vi "PS_SET_VOLTAGE.vi"(0 "VISA resource name":refnum<visa-resource-name>, 1 "SEL_PS":string(combo), 2 "Skip(T)":bool, 11 "error in (no error)":errorcluster {"code" format="%.0x"}, 12 "Use Channel":bool[](array[boolean])=[TRUE, FALSE, FALSE, FALSE], 14 "Voltage Set":sgl[](array[numeric])) -> (4 "VISA resource name out":refnum<visa-resource-name>, 15 "error out":errorcluster {"code" format="%.0x"})   [LabVIEW 2018]
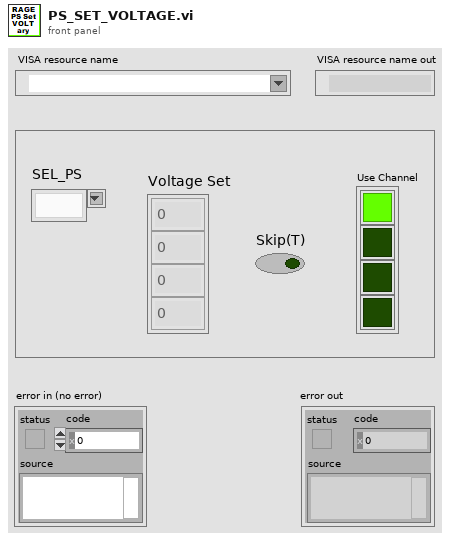
[diagram p1: front panel]
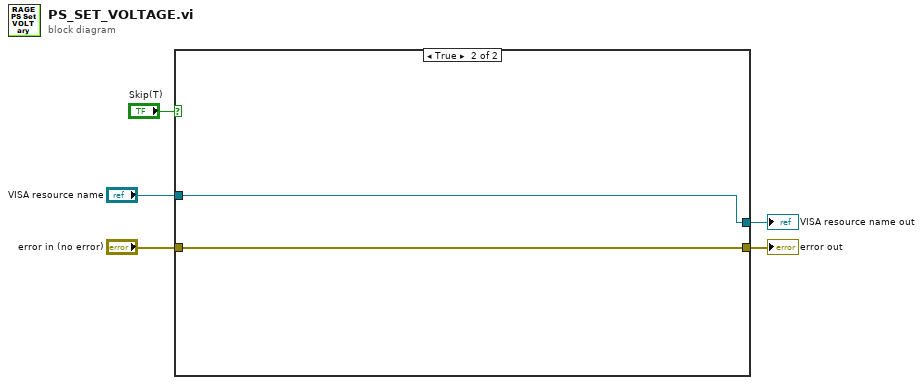
[diagram p0: block diagram]
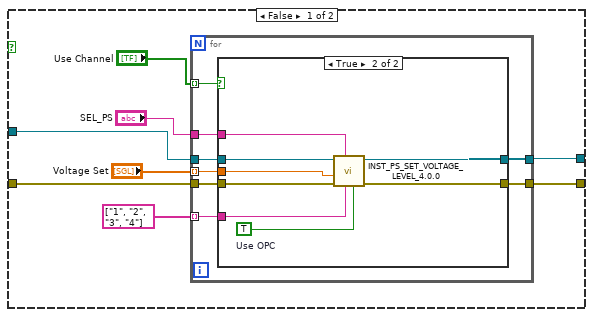
[diagram p2: hidden frame]
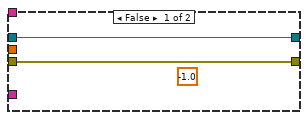
[diagram p3: hidden frame]
diagram:
  n1 = case shown="True" "Skip(T)" {
    tunnel: "error in (no error)" -> [w12 w32]
    tunnel: [w11 w32] -> w4
    tunnel: "VISA resource name" -> [w9 w33]
    tunnel: [w7 w33] -> w2
    frame False {
      n2 = for {
        tunnel: string[] ["1", "2", "3", "4"] -> [w21] mode=indexing
        tunnel: w12 -> [w20]
        tunnel: [w19] -> w11
        tunnel: "Use Channel" -> [w18] mode=indexing
        tunnel: w9 -> [w17]
        tunnel: "Voltage Set" -> [w16] mode=indexing
        tunnel: [w15] -> w7
        tunnel: "SEL_PS" -> [w14]
        n3 = case shown="True" w18 {
          tunnel: w21 -> [_ w27]
          tunnel: w20 -> [w23 w29]
          tunnel: [w23 w25] -> w19
          tunnel: w17 -> [w22 w30]
          tunnel: w16 -> [_ w31]
          tunnel: [w22 w24] -> w15
          tunnel: w14 -> [_ w28]
          frame False {
            (unwired) -1.0 ("Measurement")
          }
          frame True {
            w26 = TRUE  # Use OPC
            n4 = call "INST_PS_SET_VOLTAGE_LEVEL_4.0.0.vi"("Use OPC(T)"=w26, "Instrument Select (Output 1)"=w27, "SEL_PS"=w28, "error in (no error)"=w29, "Voltage (0.0)"=w31, "VISA session"=w30) -> ("error out"=w25:errorcluster, "dup VISA session"=w24:refnum<visa-resource-name>)  [unwired: 4 in]
          }
        }
      }
    }
    frame True {
    }
  }
  "error out" <- w4
  "VISA resource name out" <- w2
